vi "CreateTheory.vi"(5 "Theory In":refnum<class "Theory.lvclass">, 8 "error in (no error)":errorcluster, 9 "Control Data":map{string, variant}(c390), 10 "Data Name (\"\")":string, 11 "VI Refnum":refnum<vi>) -> (0 "error out":errorcluster, 3 "Theory":refnum<class "Theory.lvclass">)   [LabVIEW 2019, in "Theory.lvclass"]
uses:
  Theory.lvclass
  Theory.lvclass/Theory.ctl
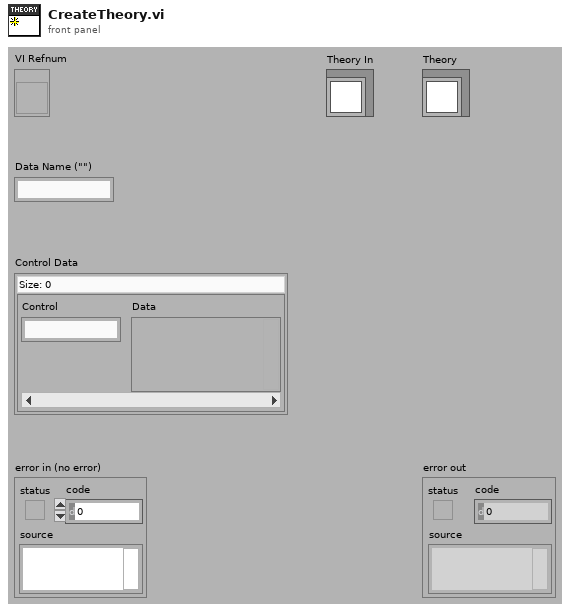
[diagram p1: front panel]
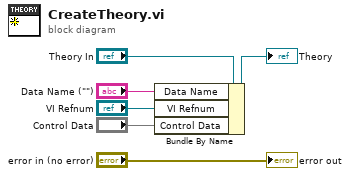
[diagram p0: block diagram]
diagram:
  n1 = Bundle By Name(cluster="Theory In", "Data Name"="Data Name (\"\")", "VI Refnum"="VI Refnum", "Control Data"="Control Data") -> (→"Theory":refnum<class "Theory.lvclass">)
  "error out" <- "error in (no error)"
